vi "DiffDriveSim_GetAllEncoderInx.vi"() -> (3 "All Encoder Inx":T1[](array[typedef]))   [LabVIEW 2019]
uses:
  <vilib>/Rock Robotics/SystemInterfaces/Encoder/FPGA_EncoderIdx.ctl
panel:
  in  "EncoderIndex":T1
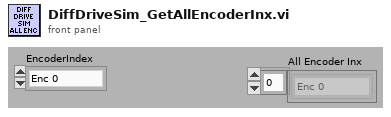
[diagram p1: front panel]
types:
  T1 = typedef "FPGA_EncoderIdx.ctl" = enum8{"Enc 0", "Enc 1", "Enc 2", "Enc 3", "Enc 4", "Enc 5", "Enc 6", "Enc 7", "Invalid"}
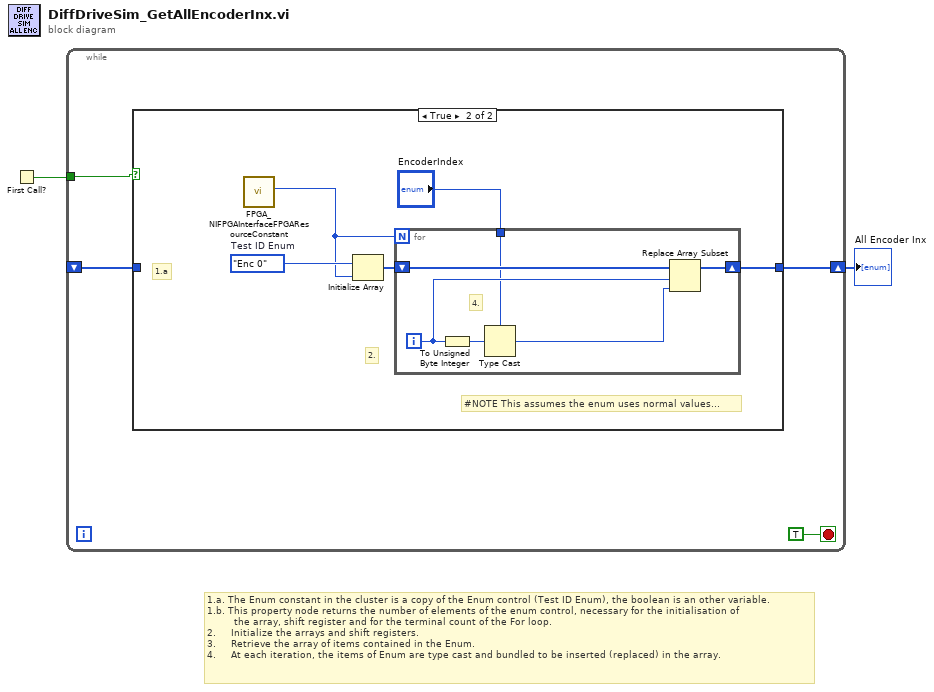
[diagram p0: block diagram]
diagram:
  # "1.a. The Enum constant in the cluster is a copy of the Enum control (Test ID Enum), the boolean is an other variable.\n1.b. This property node returns the number of elements of the enum control, necessary for the initialisation of \n         the array, shift register and for the terminal count of the For loop.\n2.     Initialize the arrays and shift registers.\n3.     Retrieve the array of items contained in the Enum.\n4.     At each iteration, the items of Enum are type cast and bundled to be inserted (replaced) in the array."
  n1 = First Call?() -> (First Call?: T/F=w2:bool)
  n2 = while {
    shift-right: [w6] -> w1
    shift-left: _ -> [w3]
    tunnel: w2 -> [w4]
    stop <- TRUE stop-if-true
    n3 = case shown="True" w4 {
      tunnel: [w7 w10] -> w6
      tunnel: w3 -> [w7 _]
      frame False {
      }
      frame True {
        w9 = FPGA_EncoderIdx."Enc 0"  # Test ID Enum
        # "#NOTE This assumes the enum uses normal values..."
        # "2."
        # "1.a"
        n4 = call <vilib>:"FPGA_NIFPGAInterfaceFPGAResourceConstant.vi"() -> ("NumberOfEncoders"=w8:u32)  [unwired: 11 out]
        n5 = Initialize Array(w9, w8) -> (w12:T1[])
        n6 = for {
          N: w8 -> [_]
          shift-right: [w17] -> w10
          shift-left: w12 -> [w18]
          tunnel: "EncoderIndex" -> [w14]
          i -> [w16]
          # "4."
          n7 = To Unsigned Byte Integer(number=w16) -> (unsigned 8bit integer=w15:u8)
          n8 = Type Cast(type=w14, x=w15) -> (*(type *) &x=w13:T1)
          n9 = Replace Array Subset(array=w18, new element=w13, index=w16) -> (w17:T1[])
        }
      }
    }
  }
  "All Encoder Inx" <- w1
